vi "EndTestSuite.vi"(8 "error in (no error)":errorcluster, 10 "TestSuite":refnum<class "TestSuite.lvclass">, 11 "FakeTestListener in":refnum<class "FakeTestListener.lvclass">) -> (0 "error out":errorcluster, 3 "FakeTestListener out":refnum<class "FakeTestListener.lvclass">)   [LabVIEW 2017, in "TestResultTest.lvlib" / "Support.lvlib" / "FakeTestListener.lvclass"]
doc: "A test suite ended."
uses:
  FakeTestListener.lvclass
  TestSuite/TestSuite.lvclass
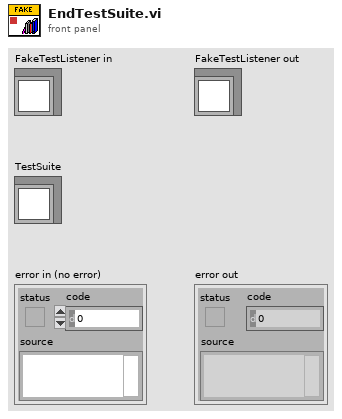
[diagram p1: front panel]
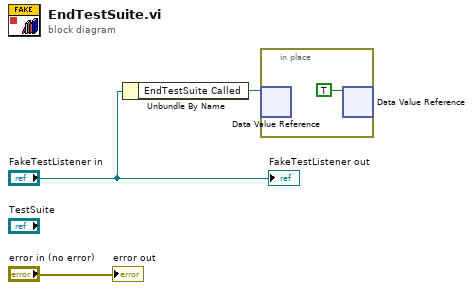
[diagram p0: block diagram]
diagram:
  n1 = Unbundle By Name("FakeTestListener in") -> ("EndTestSuite Called"=w2:refnum<data-value>)
  n2 = in-place {
    n3 = in-place-dvr #1(w2) -> ()  [unwired: 2 out]
    n4 = in-place-dvr #1(TRUE ("data value")) -> ()  [unwired: 2 out]
  }
  "error out" <- "error in (no error)"
  "FakeTestListener out" <- "FakeTestListener in"
